vi "testStringNotIncluded.vi"(9 "haystack":string, 10 "needle":string) -> (0 "error out":errorcluster)   [LabVIEW 2017, in "Assertion.Tests.lvlib" / "AssertStringContainsStringIgnoringCase.lvlib"]
uses:
  AssertStringContainsStringIgnoringCase.lvlib
  Assertion/Assertion.lvlib
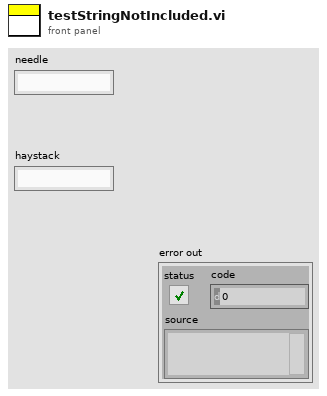
[diagram p1: front panel]
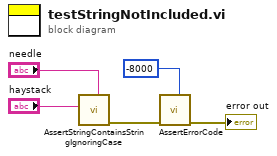
[diagram p0: block diagram]
diagram:
  n1 = call "AssertStringContainsStringIgnoringCase.vi"("Needle"="needle", "Haystack"="haystack") -> ("error out"=w2:errorcluster)  [unwired: 9 in]
  n2 = call "AssertErrorCode.vi"("Expected"=-8000, "error in (no error)"=w2) -> ("error out"=→"error out":errorcluster)  [unwired: 9 in]
